vi "Render.vi"(11 "Blob in":refnum<class "Blob.lvclass">) -> (2 "image":picture, 3 "Blob out":refnum<class "Blob.lvclass">)   [LabVIEW 2019, in "Blob.lvclass"]
doc: "Draw the image of the blob as a filled rectangle in a picture indicator."
uses:
  Blob.lvclass
  Blob.lvclass/Blob.ctl
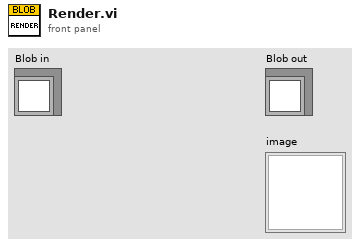
[diagram p1: front panel]
types:
  T1 = typedef "LVRectTypeDef.ctl" = cluster{"Left":i16, "Top":i16, "Right":i16, "Bottom":i16}
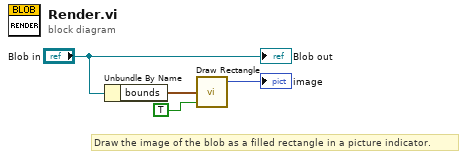
[diagram p0: block diagram]
diagram:
  # "Draw the image of the blob as a filled rectangle in a picture indicator."
  n1 = Unbundle By Name("Blob in") -> ("bounds"=w3:T1)
  n2 = call <vilib>:"Draw Rectangle.vi"("rect"=w3, "fill?(F)"=TRUE) -> ("new picture"=→"image":picture)  [unwired: 7 in]
  "Blob out" <- "Blob in"
